vi "ReadModule.vi"(9 "Transmit Frame in":T1={"timestamp high"=0, "timestamp low"=0, "identifier"=0, "type"=enum."Data Frame", "info A"=0, "info B"=0, "data length"=0, "data"=[0, 0, 0, 0, 0, 0, 0, 0]}, 10 "Numeric":i32, 11 "Numeric 2":i32) -> (3 "Transmit Frame out":T1={"timestamp high"=0, "timestamp low"=0, "identifier"=0, "type"=enum."Data Frame", "info A"=0, "info B"=0, "data length"=0, "data"=[0, 0, 0, 0, 0, 0, 0, 0]})   [LabVIEW 2016]
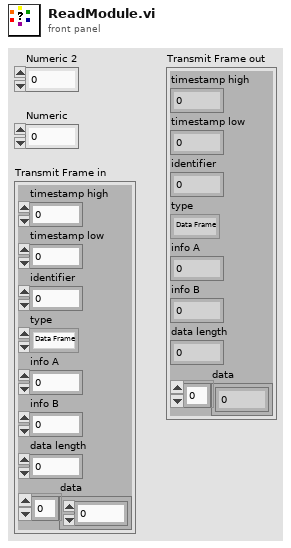
[diagram p1: front panel]
types:
  T1 = cluster{"timestamp high":u32, "timestamp low":u32, "identifier":u32, "type":enum8{"Data Frame", "Remote Frame", "(reserved)", "(reserved) ", "(reserved)  ", "(reserved)   ", "Bus Error", "Transceiver Fault"}, "info A":u8, "info B":u8, "data length":u8, "data":u8[]}
  T2 = enum8{"Data Frame", "Remote Frame", "(reserved)", "(reserved) ", "(reserved)  ", "(reserved)   ", "Bus Error", "Transceiver Fault"}
  T3 = cluster{"data[0]":u8, "data[1]":u8, "data[2]":u8, "data[3]":u8, "data[4]":u8, "data[5]":u8, "data[6]":u8, "data[7]":u8, "data[8]":u8}
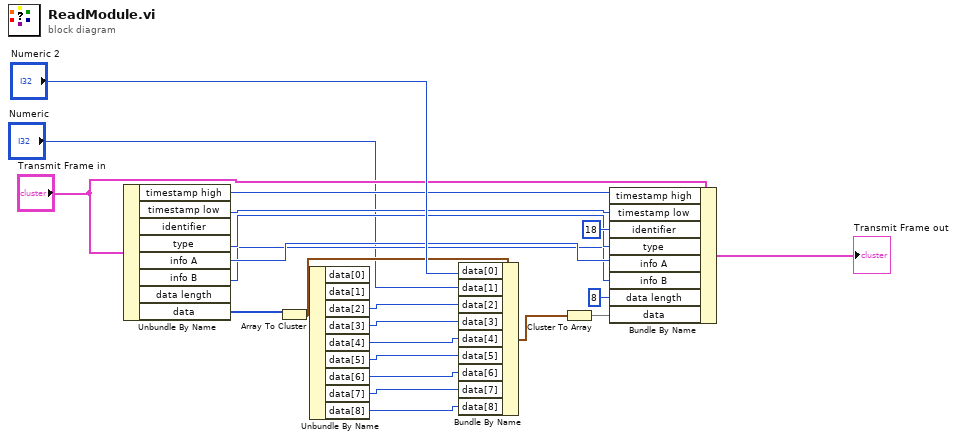
[diagram p0: block diagram]
diagram:
  n1 = Unbundle By Name("Transmit Frame in") -> ("timestamp high"=w9:u32, "timestamp low"=w8:u32, "type"=w6:T2, "info A"=w5:u8, "info B"=w4:u8, "data"=w3:u8[])  [unwired: 2 out]
  n2 = Array To Cluster(array=w3) -> (cluster=w13:T3)
  n3 = Unbundle By Name(w13) -> ("data[2]"=w1:u8, "data[3]"=w15:u8, "data[4]"=w16:u8, "data[5]"=w17:u8, "data[6]"=w18:u8, "data[7]"=w19:u8, "data[8]"=w20:u8)  [unwired: 2 out]
  n4 = Bundle By Name(cluster=w13, "data[0]"="Numeric 2", "data[1]"="Numeric", "data[2]"=w1, "data[3]"=w15, "data[4]"=w16, "data[5]"=w17, "data[6]"=w18, "data[7]"=w19, "data[8]"=w20) -> (w14:T3)
  n5 = Cluster To Array(cluster=w14) -> (array=w21:u8[])
  n6 = Bundle By Name(cluster="Transmit Frame in", "timestamp high"=w9, "timestamp low"=w8, "identifier"=u32 18, "type"=w6, "info A"=w5, "info B"=w4, "data length"=u8 8, "data"=w21) -> (→"Transmit Frame out":T1)
